vi "fifodebug.vi"() -> ()   [LabVIEW 2013]
panel:
  out "DMA Write Timeout":bool
  out "Number of Elements to Write Host DMA":u32
  out "Number of Elements to Read Cam Data":u32
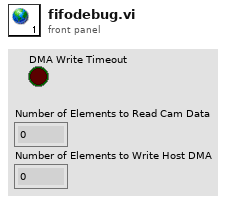
[diagram p1: front panel]
diagram:
